vi "KE2260B Configure Circuit Breaker.vi"(8 "error in (no error)":errorcluster, 10 "Circuit Breaker(F: Disable)":bool, 11 "VISA resource name":refnum<visa-resource-name>) -> (0 "error out":errorcluster, 3 "VISA resource name out":refnum<visa-resource-name>)   [LabVIEW 2009, in "Keithley 2260B.lvlib"]
doc: "Enables/Disables the power switch trip (circuit breaker) when the OVP or OCP protection settings are tripped."
uses:
  <instrlib>/Keithley 2260B/Keithley 2260B.lvlib
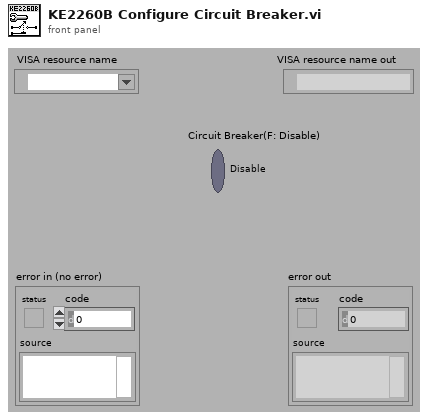
[diagram p1: front panel]
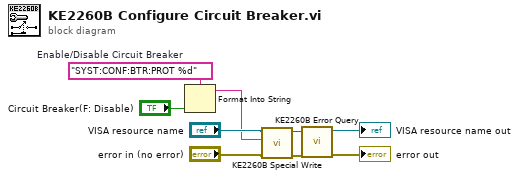
[diagram p0: block diagram]
diagram:
  w6 = "SYST:CONF:BTR:PROT %d"  # Enable/Disable Circuit Breaker
  n1 = Format Into String(format string=w6, "Circuit Breaker(F: Disable)") -> (resulting string=w1:string)  [unwired: 2 in, 1 out]
  n2 = call <instrlib>:"KE2260B Special Write.vi"("error in (no error)"="error in (no error)", "Write Buffer (\"\")"=w1, "VISA session"="VISA resource name") -> ("error out"=w5:errorcluster, "dup VISA session"=w4:refnum<visa-resource-name>)  [unwired: 6 in, 1 out]
  n3 = call <instrlib>:"KE2260B Error Query.vi"("error in (no error)"=w5, "VISA resource name"=w4) -> ("error out"=→"error out":errorcluster, "VISA resource name out"=→"VISA resource name out":refnum<visa-resource-name>)  [unwired: 6 in, 2 out]
